vi "GetTimactiveChannelNumber.vi"(2 "error in (no error)":errorcluster, 3 "Timing Channel Settings":T1[](array[typedef]) {"FrontPanelTime" format="%.3p"; "Pulse width (s)" format="%.3p"; "Delay (s)" format="%.3p"}) -> (0 "error out":errorcluster, 1 "Numeric":i16)   [LabVIEW 2013]
uses:
  Controls/TimingChannelSettings.ctl
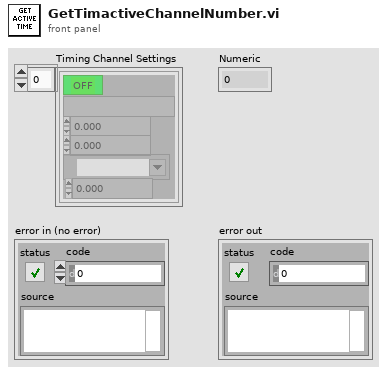
[diagram p1: front panel]
types:
  T1 = typedef "TimingChannelSettings.ctl" = cluster{"Delay (s)":dbl, "Pulse width (s)":dbl, "Active":bool, "Channel Name":string, "counter":tag, "FrontPanelTime":dbl}
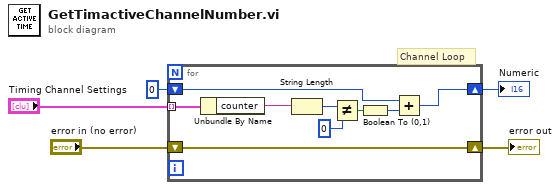
[diagram p0: block diagram]
diagram:
  # "Channel Loop"
  n1 = for {
    shift-right: [w14] -> w2
    shift-left: "error in (no error)" -> [w14]
    shift-right: [w8] -> w5
    shift-left: i16 0 -> [w9]
    tunnel: "Timing Channel Settings" -> [w7] mode=indexing
    n2 = Unbundle By Name(w7) -> ("counter"=w6:tag)
    n3 = String Length(string=w6) -> (length=w12:i32)
    n4 = Not Equal?(x=w12, y=0) -> (x != y?=w11:bool)
    n5 = Boolean To (0,1)(Boolean=w11) -> (0, 1=w10:i16)
    n6 = Add(x=w9, y=w10) -> (x+y=w8:i16)
  }
  "Numeric" <- w5
  "error out" <- w2
